vi "LabViewProject.vi"() -> ()   [LabVIEW 2024]
uses:
  <vilib>/Utility/error.llb/Trim Whitespace One-Sided.vi
  <vilib>/Instr/_visa.llb/VISA Configure Serial Port (Instr).vi
  <vilib>/Utility/file.llb/Read Delimited Spreadsheet (string).vi
  <vilib>/Utility/file.llb/Write Delimited Spreadsheet (string).vi
panel:
  in  "Voeg nieuwe kaart toe":bool
  out "all rows":string[][](array[string])
  in  "file path input":path
  in  "stop":bool
  out "serialCom":string
  in  "Port":refnum<visa-resource-name>
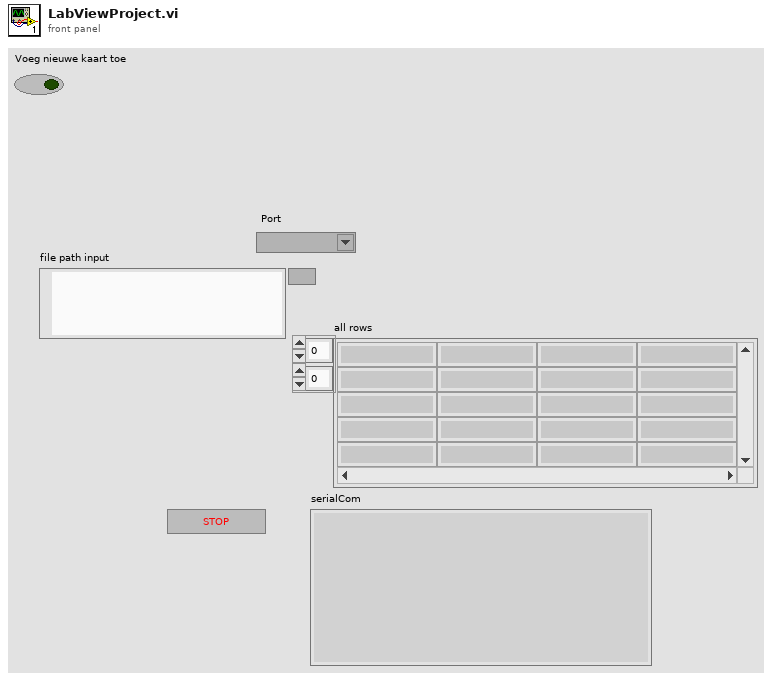
[diagram p1: front panel]
types:
  T1 = enum16{"initialize", "update_array", "checking_rfid", "access_granted", "add_new_rfid"}
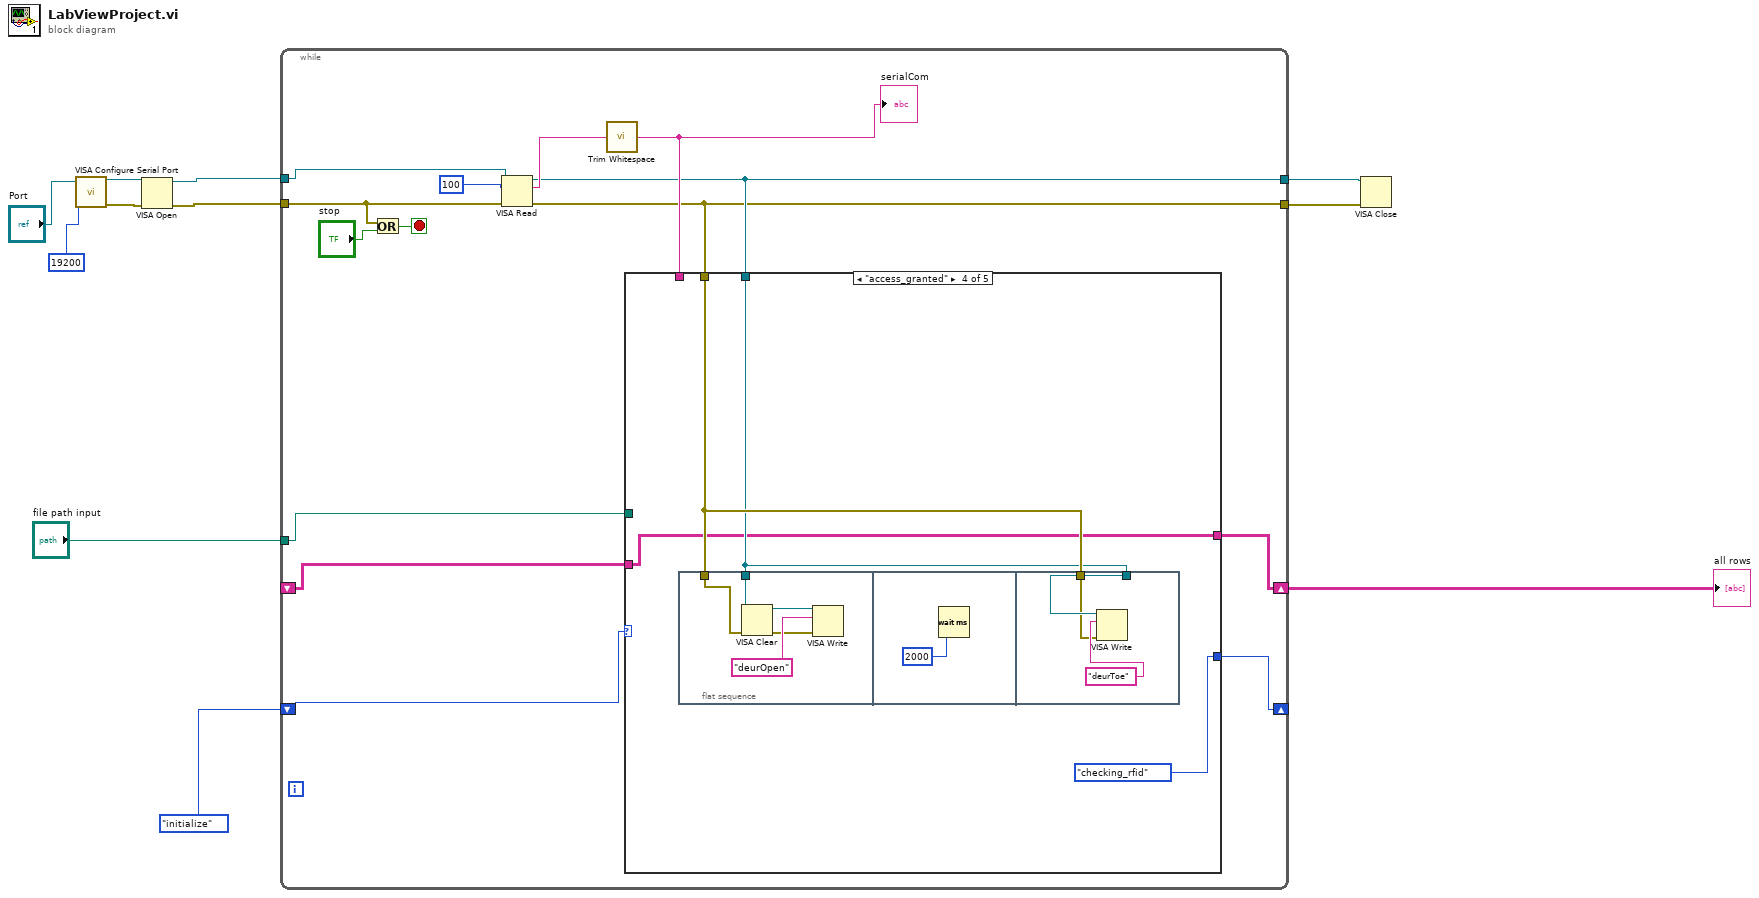
[diagram p0: block diagram]
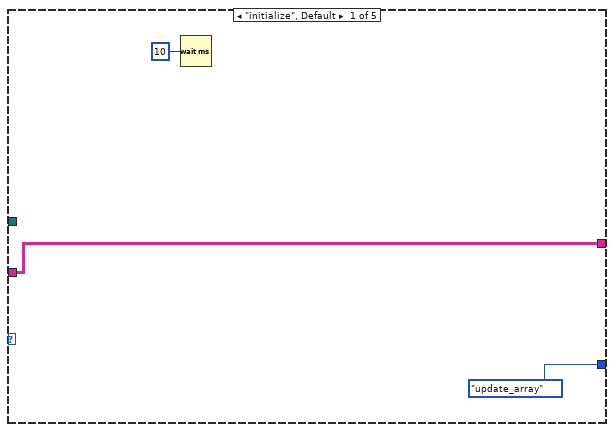
[diagram p2: hidden frame]
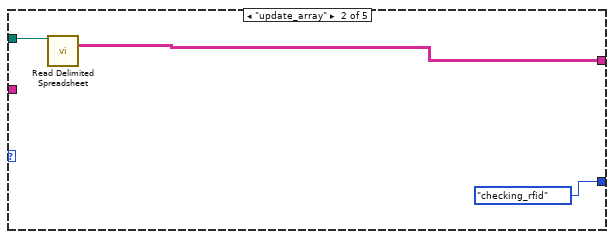
[diagram p3: hidden frame]
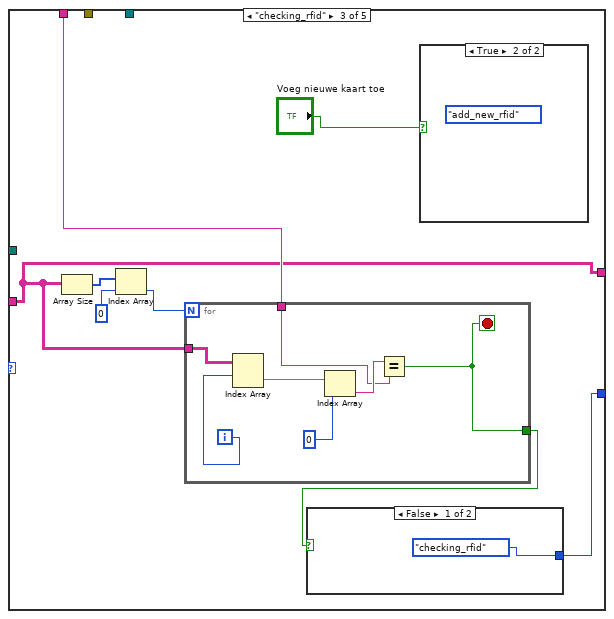
[diagram p4: hidden frame]
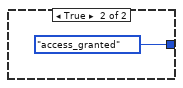
[diagram p6: hidden frame]
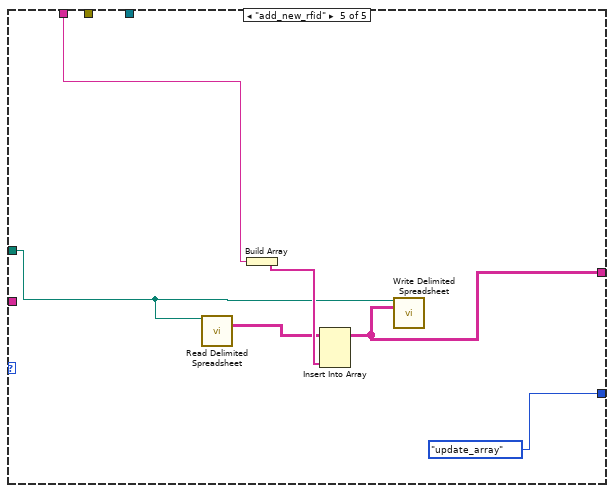
[diagram p7: hidden frame]
diagram:
  n1 = call-poly "VISA Configure Serial Port"("VISA resource name"="Port", "baud rate (9600)"=u32 19200) -> ("VISA resource name out"=w6:refnum<visa-resource-name>, "error out"=w5:errorcluster)  [unwired: 12 in]
  n2 = VISA Open(error in (no error)=w5, VISA resource name=w6) -> (VISA resource name=w8:refnum<visa-resource-name>, error out=w7:errorcluster)  [unwired: 3 in]
  n3 = while {
    tunnel: w7 -> [w24]
    tunnel: w8 -> [w23]
    tunnel: [w13] -> w10
    tunnel: [w12] -> w9
    tunnel: "file path input" -> [w17]
    shift-right: [w18] -> _
    shift-left: T1."initialize" -> [w19]
    shift-right: [w16] -> w1
    shift-left: _ -> [w15]
    stop <- w25 stop-if-true
    n4 = Or(x=w24, y="stop") -> (x .or. y?=w25:bool)
    n5 = VISA Read(VISA resource name=w23, byte count=u32 100, error in (no error)=w24) -> (VISA resource name out=w13:refnum<visa-resource-name>, read buffer=w20:string, error out=w12:errorcluster)  [unwired: 1 out]
    n6 = call <vilib>:"Trim Whitespace.vi"("string"=w20) -> ("trimmed string"=w14:string)  [unwired: 1 in]
    "serialCom" <- w14
    n7 = case shown="\"access_granted\"" w19 {
      tunnel: [T1."update_array" T1."checking_rfid" w34 T1."checking_rfid" T1."update_array"] -> w18
      tunnel: w17 -> [_ w31 _ _ w64]
      tunnel: [w27 w30 w32 w49 w62] -> w16
      tunnel: w15 -> [w27 _ w32 w49 _]
      tunnel: w14 -> [_ _ w36 _ w65]
      tunnel: w12 -> [_ _ _ w52 _]
      tunnel: w13 -> [_ _ _ w51 _]
      frame "initialize", Default {
        n8 = Wait (ms)(milliseconds to wait=u32 10 ("millisecond multiple")) -> ()  [unwired: 1 out]
      }
      frame "update_array" {
        n9 = call-poly <vilib>:"Read Delimited Spreadsheet.vi"("file path (dialog if empty)"=w31) -> ("all rows"=w30:string[][])  [unwired: 9 in, 5 out]
      }
      frame "checking_rfid" {
        n10 = Array Size(array=w32) -> (size(s)=w38:i32[])
        n11 = Index Array(array=w38, index=0) -> (element=w39:i32)
        n12 = for {
          N: w39 -> [_]
          tunnel: w36 -> [w43]
          tunnel: w32 -> [w48]
          tunnel: [w42] -> w35
          i -> [w44]
          stop <- w42 stop-if-true
          n13 = Index Array(array=w48, index (row)=w44) -> (element=w45:string[])  [unwired: 1 in]
          n14 = Index Array(array=w45, index=0) -> (element=w47:string)
          n15 = Equal?(x=w47, y=w43) -> (x = y?=w42:bool)
        }
        n16 = case shown="False" w35 {
          tunnel: [T1."checking_rfid" T1."access_granted"] -> w34
          frame False {
          }
          frame True {
          }
        }
        n17 = case shown="True" "Voeg nieuwe kaart toe" {
          frame False {
          }
          frame True {
            (unwired) T1."add_new_rfid"
          }
        }
      }
      frame "access_granted" {
        n18 = flat-sequence {
          tunnel: w52 -> [w56]
          tunnel: w51 -> [w55]
          tunnel: w51 -> [w60]
          tunnel: w52 -> [w59]
          frame #0 {
            n19 = VISA Clear(VISA resource name=w55, error in (no error)=w56) -> (VISA resource name out=w54:refnum<visa-resource-name>, error out=w53:errorcluster)
            n20 = VISA Write(VISA resource name=w54, write buffer="deurOpen", error in (no error)=w53) -> ()  [unwired: 3 out]
          }
          frame #1 {
            n21 = Wait (ms)(milliseconds to wait=u32 2000) -> ()  [unwired: 1 out]
          }
          frame #2 {
            n22 = VISA Write(VISA resource name=w60, write buffer="deurToe", error in (no error)=w59) -> ()  [unwired: 3 out]
          }
        }
      }
      frame "add_new_rfid" {
        n23 = call-poly <vilib>:"Read Delimited Spreadsheet.vi"("file path (dialog if empty)"=w64) -> ("all rows"=w66:string[][])  [unwired: 9 in, 5 out]
        n24 = Build Array(w65) -> (w67:string[])
        n25 = Insert Into Array(array=w66, new element=w67) -> (w62:string[][])  [unwired: 2 in]
        n26 = call-poly <vilib>:"Write Delimited Spreadsheet.vi"("file path (dialog if empty)"=w64, "2D data"=w62) -> ()  [unwired: 12 in, 2 out]
      }
    }
  }
  "all rows" <- w1
  n27 = VISA Close(VISA resource name=w10, error in (no error)=w9) -> ()  [unwired: 1 out]
